vi "Add.vi"(8 "error in (no error)":errorcluster, 9 "Style":T1, 10 "Name":string, 11 "FSM.Annotation in":refnum<class "FSM.Annotation.lvclass">) -> (0 "error out":errorcluster, 2 "Changed?":bool, 3 "FSM.Annotation out":refnum<class "FSM.Annotation.lvclass">)   [LabVIEW 2015, in "FSM.Annotation.lvclass"]
uses:
  FSM.Annotation.lvclass
  Annotation Style.ctl
  FSM.Annotation.lvclass/FSM.Annotation.ctl
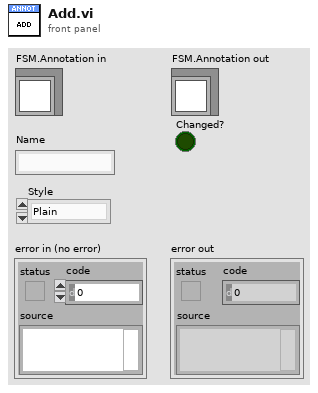
[diagram p1: front panel]
types:
  T1 = typedef "FSM.Annotation.lvclass/Annotation Style.ctl" = enum16{"Plain", "On", "Off", "On-Off"}
  T2 = cluster{"Name":string, "Style":enum16{"Plain", "On", "Off", "On-Off"}}[]
  T3 = cluster{"Name":string, "Style":enum16{"Plain", "On", "Off", "On-Off"}}
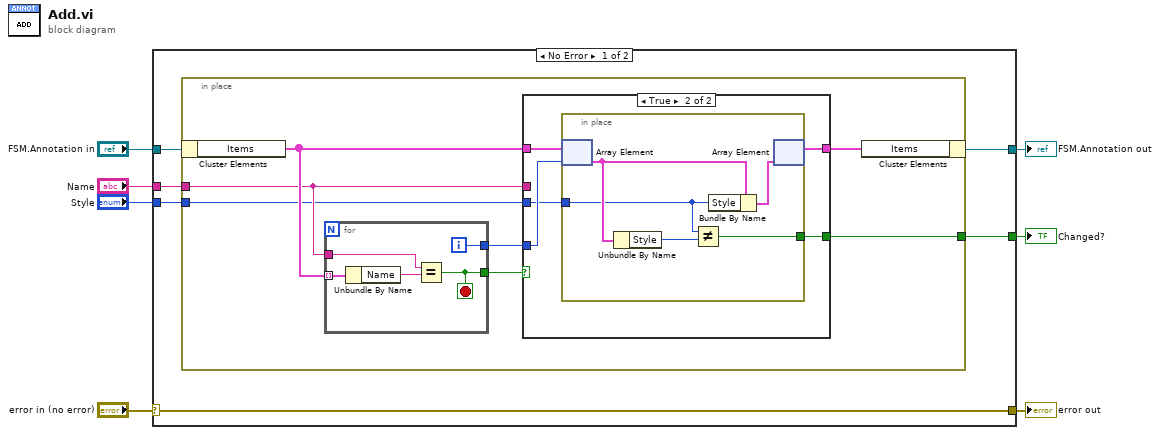
[diagram p0: block diagram]
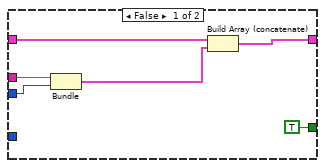
[diagram p2: hidden frame]
diagram:
  n1 = case shown="No Error" "error in (no error)" {
    selector: "error in (no error)" -> [w13 w43]
    tunnel: [w13 w43] -> w6
    tunnel: [w11 w42] -> w4
    tunnel: "FSM.Annotation in" -> [w12 w42]
    tunnel: "Name" -> [w10 _]
    tunnel: "Style" -> [w9 _]
    tunnel: [w8 _] -> w1
    frame No Error {
      n2 = in-place {
        in-place-border: w10 -> [w17]
        in-place-border: w9 -> [w16]
        in-place-border: [w14] -> w8
        n3 = in-place-cluster #1(w12) -> ("Items"=w18:T2)
        n4 = for {
          tunnel: w18 -> [w39] mode=indexing
          tunnel: w17 -> [w40]
          tunnel: [w38] -> w19
          tunnel: [w37] -> w20
          i -> [w37]
          stop <- w38 stop-if-true
          n5 = Unbundle By Name(w39) -> ("Name"=w41:string)
          n6 = Equal?(x=w40, y=w41) -> (x = y?=w38:bool)
        }
        n7 = case shown="True" w19 {
          tunnel: w18 -> [w26 w31]
          tunnel: w20 -> [_ w30]
          tunnel: w16 -> [w23 w29]
          tunnel: [w25 w28] -> w15
          tunnel: w17 -> [w24 _]
          tunnel: [TRUE w27] -> w14
          frame False {
            n8 = Bundle("Name"=w24, "Style"=w23) -> (w22:cluster{"Name":string, "Style":T1})  [unwired: 1 in]
            n9 = Build Array (concatenate)(w26, w22) -> (w25:cluster{"Name":string, "Style":T1}[])
          }
          frame True {
            n10 = in-place {
              in-place-border: w29 -> [w33]
              in-place-border: [w32] -> w27
              n11 = in-place-array #2(w31, w30) -> (w35:T3)
              n12 = Unbundle By Name(w35) -> ("Style"=w34:enum16{"Plain", "On", "Off", "On-Off"})
              n13 = Not Equal?(x=w33, y=w34) -> (x != y?=w32:bool)
              n14 = Bundle By Name(cluster=w35, "Style"=w33) -> (w36:T3)
              n15 = in-place-array #2(w36) -> (w28:T2)  [unwired: 1 out]
            }
          }
        }
        n16 = in-place-cluster #1("Items"=w15) -> (w11:refnum<class "FSM.Annotation.lvclass">)
      }
    }
    frame Error {
    }
  }
  "error out" <- w6
  "FSM.Annotation out" <- w4
  "Changed?" <- w1
